vi "Get line state.vi"(8 "error in (no error)":errorcluster, 10 "Line number":u8, 11 "TTL in":refnum<class "TTL.lvclass">) -> (0 "error out":errorcluster, 2 "Line state":bool, 3 "TTL out":refnum<class "TTL.lvclass">)   [LabVIEW 2011, in "TTL.lvclass"]
uses:
  TTL.lvclass
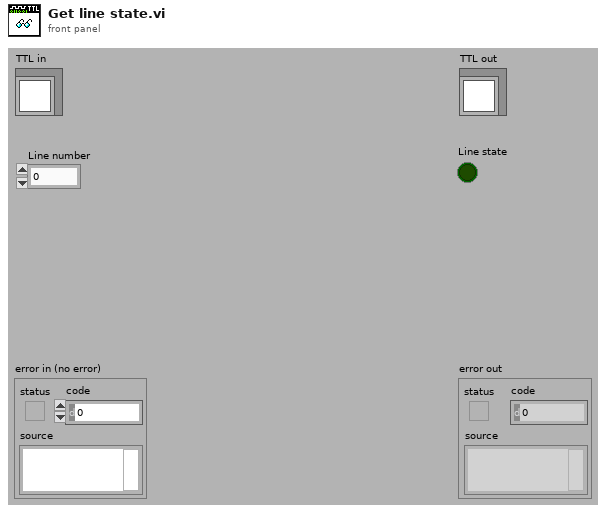
[diagram p1: front panel]
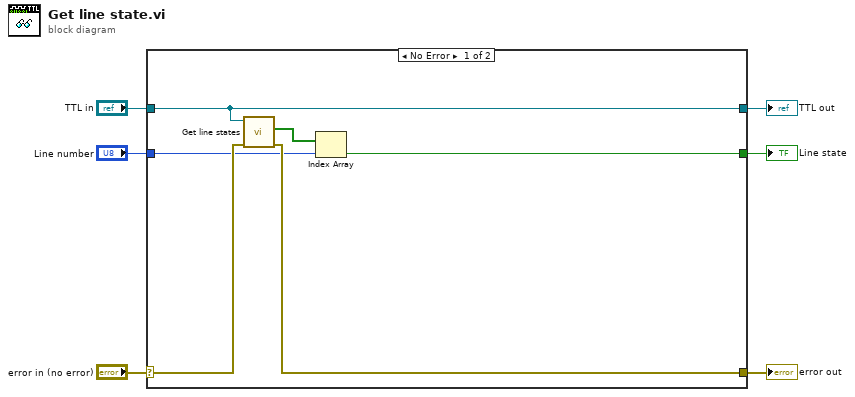
[diagram p0: block diagram]
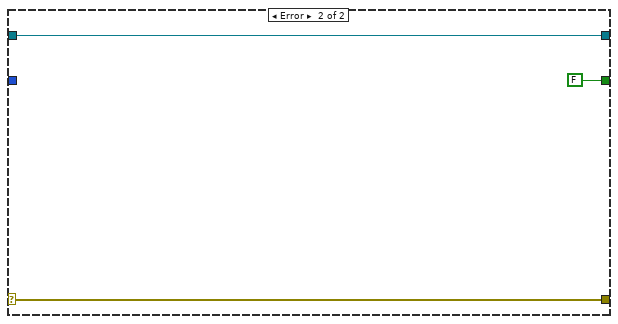
[diagram p2: hidden frame]
diagram:
  n1 = case shown="No Error" "error in (no error)" {
    selector: "error in (no error)" -> [w11 w15]
    tunnel: [w12 w15] -> w5
    tunnel: [w9 w14] -> w3
    tunnel: "TTL in" -> [w9 w14]
    tunnel: "Line number" -> [w10 _]
    tunnel: [w7 FALSE ("Boolean")] -> w1
    frame No Error {
      n2 = call "Get line states.vi"("error in (no error)"=w11, "TTL in"=w9) -> ("error out"=w12:errorcluster, "Current line states"=w8:bool[])  [unwired: 7 in, 1 out]
      n3 = Index Array(array=w8, index=w10) -> (element=w7:bool)
    }
    frame Error {
    }
  }
  "error out" <- w5
  "TTL out" <- w3
  "Line state" <- w1
